vi "Initialize Test Numbers.vi"(0 "Test Num and Bin Gen In":refnum<class "Test Number and Bin Generator.lvclass">=refnum, 11 "error in (no error)":errorcluster) -> (4 "Test Num and Bin Gen Out":refnum<class "Test Number and Bin Generator.lvclass">, 15 "error out":errorcluster)   [LabVIEW 2018, in "Test Number and Bin Generator.lvlib" / "Test Number and Bin Generator.lvclass"]
uses:
  Test Number and Bin Generator.lvclass
  Test Number and Bin Generator.lvclass/Test Number and Bin Generator.ctl
  Plugins/TestStand API Tools (TSAT).lvlibp/Evaluation Actions/Includes/Controls/TSAT Evaluation.ctl
  Plugins/TestStand API Tools (TSAT).lvlibp/Evaluation Actions/Includes/Controls/TSAT Eval SI Unit Scaling.ctl
  Plugins/TestStand API Tools (TSAT).lvlibp/Evaluation Actions/Includes/Controls/TSAT Evaluation Type.ctl
  Plugins/TestStand API Tools (TSAT).lvlibp/Evaluation Actions/TSAT Evaluation Actions.lvlib
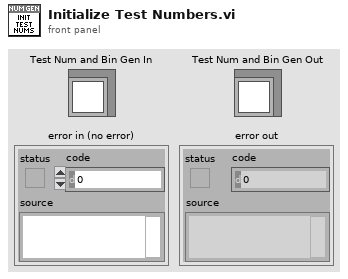
[diagram p1: front panel]
types:
  T1 = typedef "TestStand API Tools (TSAT).lvlibp/TSAT Evaluation Actions.lvlib/TSAT Evaluation.ctl" = cluster{"Test Name":string, "Pin":string, "Units":string, "SI Scaling":T2, "Test Number":i32, "Published Data Id":string, "Low Limit":dbl, "High Limit":dbl, "Export Data Location":string, "Software Bin":i64, "Evaluation Type":T3, "Test Data Source":string}
  T2 = typedef "TestStand API Tools (TSAT).lvlibp/TSAT Evaluation Actions.lvlib/TSAT Eval SI Unit Scaling.ctl" = i16
  T3 = typedef "TestStand API Tools (TSAT).lvlibp/TSAT Evaluation Actions.lvlib/TSAT Evaluation Type.ctl" = enum16{"Numeric Limit", "Pass/Fail", "None"}
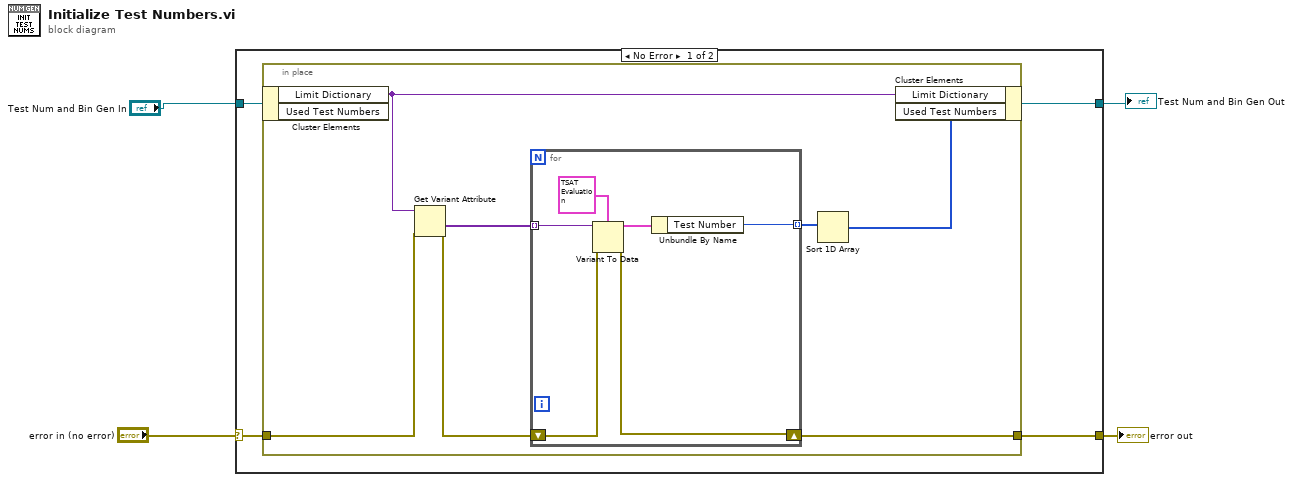
[diagram p0: block diagram]
diagram:
  n1 = case shown="No Error" "error in (no error)" {
    selector: "error in (no error)" -> [w7 w23]
    tunnel: [w8 w23] -> w4
    tunnel: [w6 w22] -> w2
    tunnel: "Test Num and Bin Gen In" -> [w5 w22]
    frame No Error {
      n2 = in-place {
        in-place-border: [w9] -> w8
        in-place-border: w7 -> [w14]
        n3 = in-place-cluster #1(w5) -> ("Limit Dictionary"=w15:variant)  [unwired: 1 out]
        n4 = Get Variant Attribute(Variant=w15, error in=w14) -> (values=w13:variant[], error out=w10:errorcluster)  [unwired: 2 in, 2 out]
        n5 = for {
          tunnel: w13 -> [w21] mode=indexing
          tunnel: [w20] -> w12 mode=indexing
          shift-right: [w16] -> w9
          shift-left: w10 -> [w17]
          n6 = Variant To Data(error in=w17, type=T1 {"Test Name"="", "Pin"="", "Units"="", "SI Scaling"=0, "Test Number"=0, "Published Data Id"="", "Low Limit"=0.0, "High Limit"=0.0, "Export Data Location"="", "Software Bin"=0, "Evaluation Type"=enum."Numeric Limit", "Test Data Source"=""} ("Evaluation"), Variant=w21) -> (data=w18:T1, error out=w16:errorcluster)
          n7 = Unbundle By Name(w18) -> ("Test Number"=w20:i32)
        }
        n8 = Sort 1D Array(array=w12) -> (sorted array=w11:i32[])
        n9 = in-place-cluster #1("Limit Dictionary"=w15, "Used Test Numbers"=w11) -> (w6:refnum<class "Test Number and Bin Generator.lvclass">)
      }
    }
    frame Error {
    }
  }
  "error out" <- w4
  "Test Num and Bin Gen Out" <- w2
